vi "Control_P.vi"(1 "Posición anterior":dbl, 2 "Parar":bool, 3 "Centroide":cluster{"X Centroid":sgl, "Y Centroid":sgl}, 4 "Kp":dbl=0.02) -> (0 "Posición":dbl)   [LabVIEW 2014]
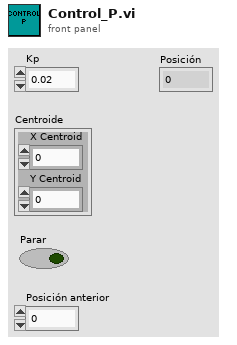
[diagram p1: front panel]
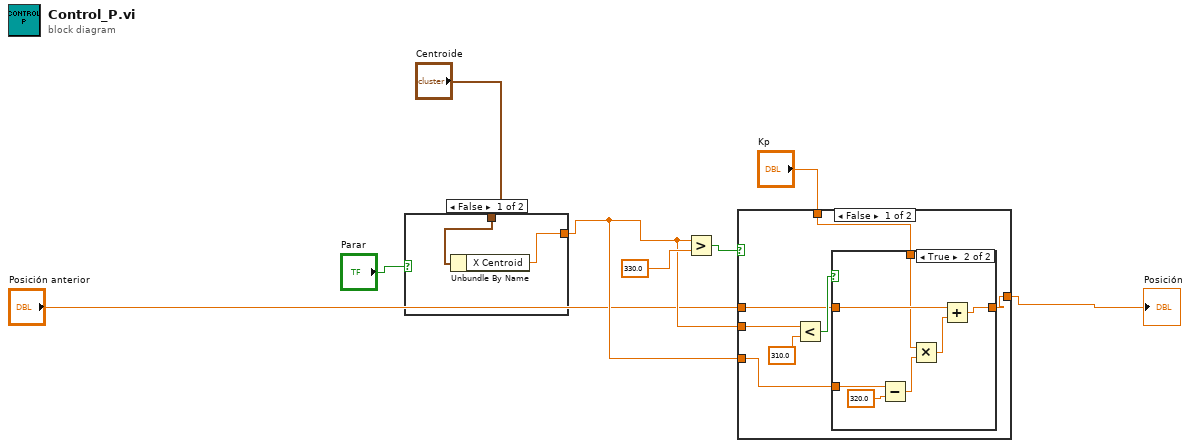
[diagram p0: block diagram]
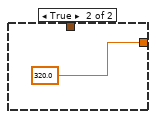
[diagram p2: hidden frame]
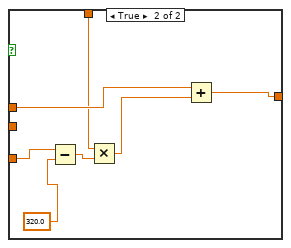
[diagram p4: hidden frame]
diagram:
  n1 = case shown="False" "Parar" {
    tunnel: "Centroide" -> [w10 _]
    tunnel: [w9 320.0] -> w5
    frame False {
      n2 = Unbundle By Name(w10) -> ("X Centroid"=w9:sgl)
    }
    frame True {
    }
  }
  n3 = Greater?(x=w5, y=sgl 330.0) -> (0:w1:bool)
  n4 = case shown="False" w1 {
    tunnel: [w18 w32] -> w3
    tunnel: "Posición anterior" -> [w15 w33]
    tunnel: w5 -> [w16 _]
    tunnel: w5 -> [w13 w29]
    tunnel: "Kp" -> [w12 w27]
    frame False {
      n5 = Less?(x=w16, y=310.0) -> (x < y?=w17:bool)
      n6 = case shown="True" w17 {
        tunnel: [w19 w26] -> w18
        tunnel: w15 -> [w19 w23]
        tunnel: w13 -> [_ w24]
        tunnel: w12 -> [_ w20]
        frame False {
        }
        frame True {
          n7 = Subtract(x=w24, y=320.0) -> (x-y=w22:dbl)
          n8 = Multiply(x=w20, y=w22) -> (x*y=w21:dbl)
          n9 = Add(x=w23, y=w21) -> (x+y=w26:dbl)
        }
      }
    }
    frame True {
      n10 = Subtract(x=w29, y=320.0) -> (x-y=w31:dbl)
      n11 = Multiply(x=w27, y=w31) -> (x*y=w30:dbl)
      n12 = Add(x=w33, y=w30) -> (x+y=w32:dbl)
    }
  }
  "Posición" <- w3
